vi "PythonNode_NumpyMatmul.vi"() -> ()   [LabVIEW 2019]
doc: "This example demonstrates how to call a Python function and pass arguments as numpy arrays. It uses a python function to compute the product of two matrices."
uses:
  support/PythonVersionsEnum.ctl
panel:
  out "a*b":dbl[][](array[numeric])
  in  "b":dbl[][](array[numeric])=[[1.0, 0.0, 0.0], [0.0, 1.0, 0.0], [0.0, 0.0, 1.0]]
  in  "a":dbl[][](array[numeric])=[[1.0, 2.0, 3.0], [4.0, 5.0, 6.0], [7.0, 8.0, 9.0]]
  out "error out":errorcluster
  in  "error in (no error)":errorcluster
  in  "python version":T1
  # "Overview: Demonstrates how to call a Python function and pass arrays as numpy arrays.\nRequirements: Python 2.7 or 3.6 with the same bitness as LabVIEW with numpy installed.\nInstructions:\n1. Set the Python version to the version of Python you want to execute code in.\n2. Run the VI. You should see the result of multiplying the matrix  \"a\" by the matrix \"b\" in the indicator \"a*b\".\n3. See comments on the block diagram of this VI and in \"ExamplePythonModule.py\" for more information about how the call python node passes arguments and handles return values."
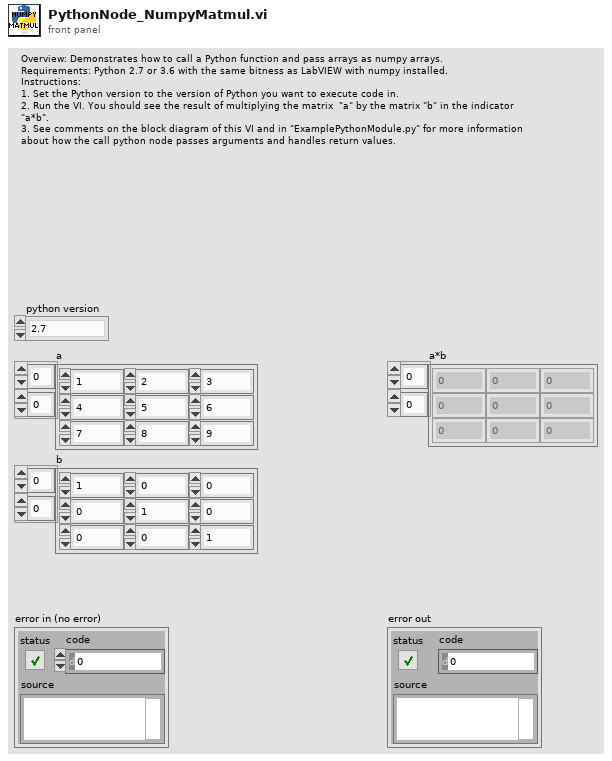
[diagram p1: front panel]
types:
  T1 = typedef "PythonVersionsEnum.ctl" = enum16{"2.7", "3.6"}
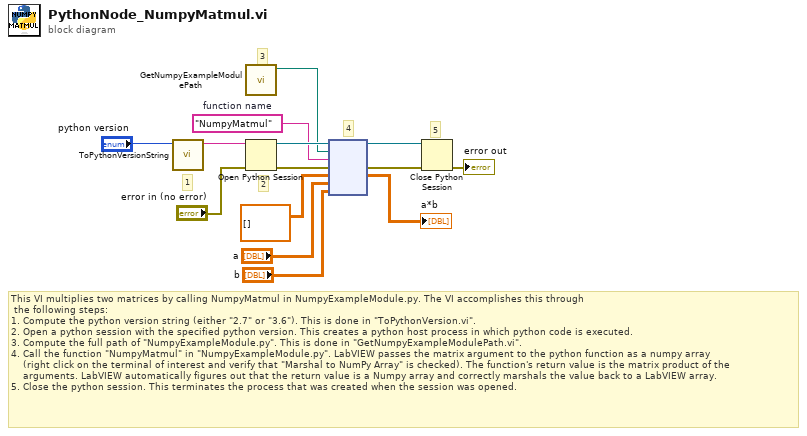
[diagram p0: block diagram]
diagram:
  w8 = "NumpyMatmul"  # function name
  # "5"
  # "4"
  # "2"
  # "3"
  # "1"
  # "This VI multiplies two matrices by calling NumpyMatmul in NumpyExampleModule.py. The VI accomplishes this through\n the following steps:\n1. Compute the python version string (either \"2.7\" or \"3.6\"). This is done in \"ToPythonVersion.vi\". \n2. Open a python session with the specified python version. This creates a python host process in which python code is executed.\n3. Compute the full path of \"NumpyExampleModule.py\". This is done in \"GetNumpyExampleModulePath.vi\".\n4. Call the function \"NumpyMatmul\" in \"NumpyExampleModule.py\". LabVIEW passes the matrix argument to the python function as a numpy array\n    (right click on the terminal of interest and verify that \"Marshal to NumPy Array\" is checked). The function's return value is the matrix product of the\n    arguments. LabVIEW automatically figures out that the return value is a Numpy array and correctly marshals the value back to a LabVIEW array.\n5. Close the python session. This terminates the process that was created when the session was opened."
  n1 = call "ToPythonVersionString.vi"("python version"="python version") -> ("python version string"=w14:string)  [unwired: 10 in]
  n2 = call "GetNumpyExampleModulePath.vi"() -> ("module path"=w9:path)  [unwired: 11 in]
  n3 = Open Python Session(python version=w14, 3:"error in (no error)") -> (session out=w11:refnum<k35>, error out=w10:errorcluster)  [unwired: 1 in]
  n4 = node(w11, w9, w8, w10, dbl[][] [] ("b"), "a", "b") -> (w7:refnum<k35>, w6:errorcluster, →"a*b":dbl[][])  [unwired: 2 in, 2 out]
  n5 = Close Python Session(session in=w7, error in=w6) -> (11:→"error out":errorcluster)
